vi "Do.vi"(8 "error in (no error)":errorcluster, 11 "_State Machine Actor in":refnum<class "_State Machine Actor.lvclass">) -> (0 "error out":errorcluster, 3 "_State Machine Actor out":refnum<class "_State Machine Actor.lvclass">)   [LabVIEW 2024, in "_State Machine Actor.lvlib" / "_State Machine Actor.lvclass"]
uses:
  _State Machine Actor.lvclass
  _State Machine Actor.lvclass/_State Machine Actor.ctl
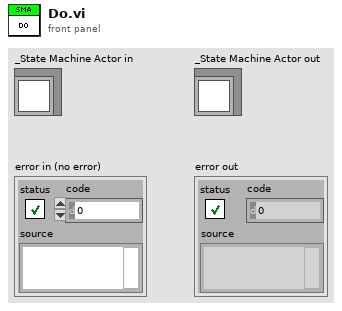
[diagram p1: front panel]
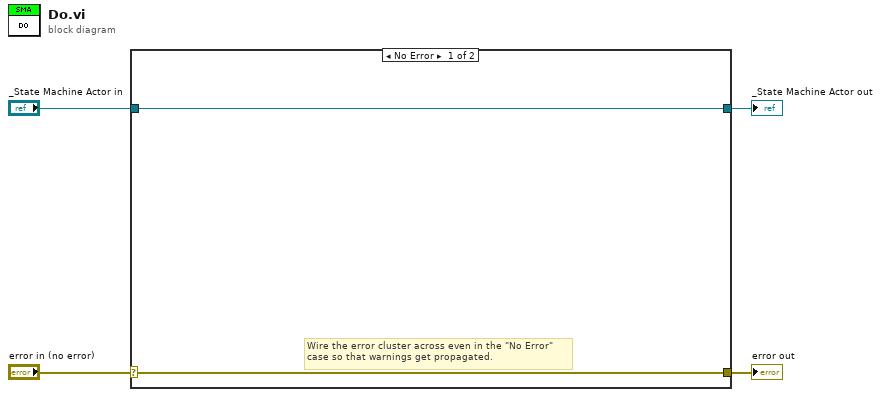
[diagram p0: block diagram]
diagram:
  n1 = case shown="No Error" "error in (no error)" {
    selector: "error in (no error)" -> [w5 w8]
    tunnel: [w5 w8] -> w3
    tunnel: [w6 w7] -> w1
    tunnel: "_State Machine Actor in" -> [w6 w7]
    frame No Error {
      # "Wire the error cluster across even in the \"No Error\"\ncase so that warnings get propagated."
    }
    frame Error {
    }
  }
  "error out" <- w3
  "_State Machine Actor out" <- w1
